vi "Print Initialization Message.vi"(8 "error in (no error)":errorcluster, 11 "Parameters":T1={"Interface Data"={"Name"="", "Unit ID"=0, "Refresh Rate"=0, "Interface Type"=enum."TCP Master", "TCP Settings"={"Address"="", "Port"=0, "Timeout"=0}, "Serial Settings"={"VISA resource name"="", "baud rate"=0, "parity (even)"=0, "flow control (none)"=0, "serial type"=enum."RTU", "Wire Mode"=-1}}, "Modbus Input Groups"=[], "Modbus Output Groups"=[], "error in (no error)"={"status"=FALSE, "code"=0, "source"=""}, "Modbus Input Engine Group Names"=[], "Modbus Output Engine Group Names"=[]} {"Interface Data"."Serial Settings"."Wire Mode" items=["Unknown"=-1, "RS485/Wire4"=0, "RS485/Wire2-EchoDTR"=1, "RS485/Wire2-CtrlDTR"=2, "RS485/Wire2-Auto"=3, "RS232/DTE"=128, "RS232/DCE"=129, "RS232/AUTO"=130]; "Interface Data"."Serial Settings"."parity (even)" items=["None", "Odd", "Even", "Mark", "Space"]; "Interface Data"."Serial Settings"."flow control (none)" items=["None", "XON/XOFF", "RTS/CTS", "XON/XOFF & RTS/CTS", "DTR/DSR", "XON/XOFF & DTR/DSR"]}) -> (0 "error out":errorcluster)   [LabVIEW 2015, in "Modbus Master Engine.lvlib"]
uses:
  Modbus Master Engine.lvlib
  Shared/Device Info.ctl
  Shared/Controls/Interface Type.ctl
  Shared/Controls/Data Model/TCP Settings.ctl
  Shared/Controls/Data Model/Serial Settings.ctl
  Bulk Data Access.ctl
  System Explorer/SubVIs/Modbus Type.ctl
  Shared/Controls/Data Model/Channel.ctl
  <vilib>/NI Veristand/Custom Device API/Custom Device Channel Type.ctl
  Shared/Controls/Data Model/Mapping.ctl
  Shared/Controls/Data Model/DataType.ctl
  <vilib>/NI Veristand/Custom Device API/Custom Device Item Ref.ctl
  <vilib>/NI VeriStand/Custom Device Tools/Custom Device Utility Library/Custom Device Utility Library.lvlib
  Shared/Modbus Master Shared.lvlib
  <vilib>/NI VeriStand/Custom Device API/Custom Device API.lvlib
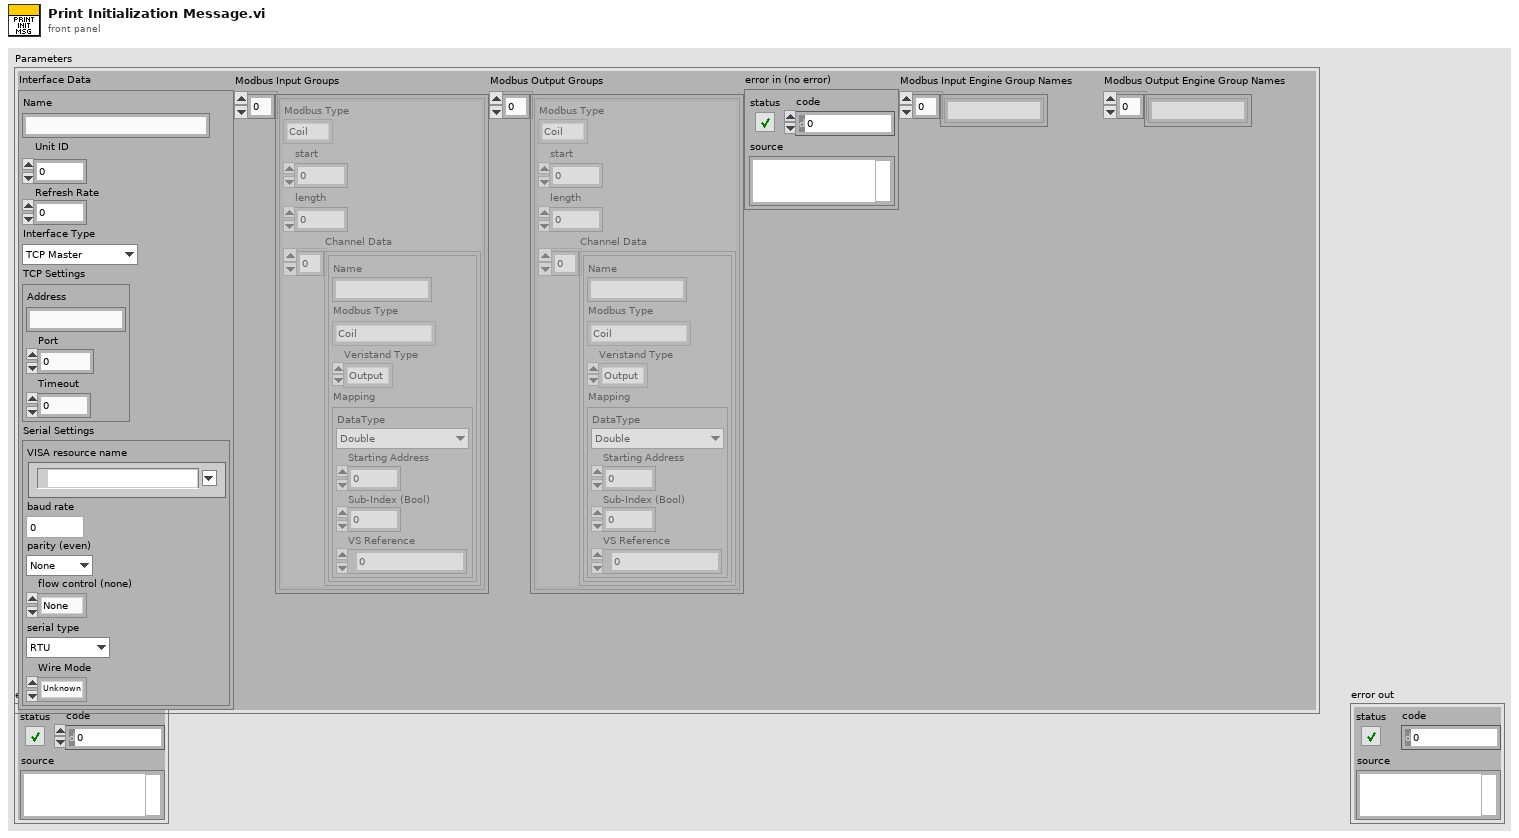
[diagram p1: front panel]
types:
  T1 = typedef "Modbus Master Shared.lvlib/Device Info.ctl" = cluster{"Interface Data":cluster{"Name":string, "Unit ID":u8, "Refresh Rate":i32, "Interface Type":T2, "TCP Settings":T3, "Serial Settings":T4}, "Modbus Input Groups":T5[], "Modbus Output Groups":T5[], "error in (no error)":errorcluster, "Modbus Input Engine Group Names":string[], "Modbus Output Engine Group Names":string[]}
  T2 = typedef "Modbus Master Shared.lvlib/Interface Type.ctl" = enum16{"TCP Master", "Serial Master", "TCP Slave", "Serial Slave"}
  T3 = typedef "Modbus Master Shared.lvlib/TCP Settings.ctl" = cluster{"Address":string, "Port":u16, "Timeout":i32}
  T4 = typedef "Modbus Master Shared.lvlib/Serial Settings.ctl" = cluster{"VISA resource name":refnum<visa-resource-name>, "baud rate":u32, "parity (even)":u16, "flow control (none)":u16, "serial type":enum16{"RTU", "ASCII"}, "Wire Mode":i16}
  T5 = typedef "Modbus Master Shared.lvlib/Bulk Data Access.ctl" = cluster{"Modbus Type":T6, "start":u16, "length":u16, "Channel Data":T7[]}
  T6 = typedef "Modbus Master Shared.lvlib/Modbus Type.ctl" = enum16{"Coil", "Discrete Input", "Holding Register", "Input Register"}
  T7 = typedef "Modbus Master Shared.lvlib/Channel.ctl" = cluster{"Name":string, "Modbus Type":T6, "Veristand Type":T8, "Mapping":T9}
  T8 = typedef "Custom Device API.lvlib/Custom Device Channel Type.ctl" = enum16{"Input", "Output"}
  T9 = typedef "Modbus Master Shared.lvlib/Mapping.ctl" = cluster{"DataType":T10, "Starting Address":u16, "Sub-Index (Bool)":u16, "VS Reference":T11}
  T10 = typedef "Modbus Master Shared.lvlib/DataType.ctl" = enum16{"Double", "Single", "I64", "I32", "I16", "I8", "U64", "U32", "U16", "U8", "Boolean"}
  T11 = typedef "Custom Device API.lvlib/Custom Device Item Ref.ctl" = u64
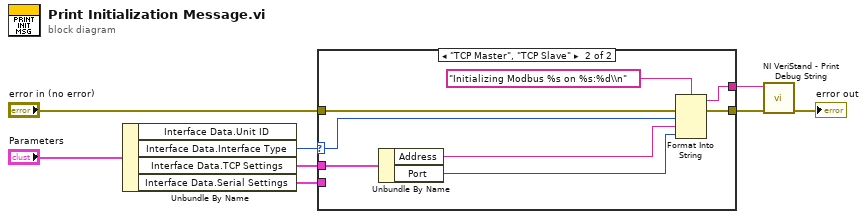
[diagram p0: block diagram]
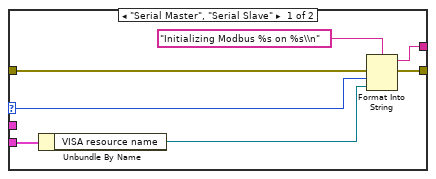
[diagram p2: hidden frame]
diagram:
  n1 = Unbundle By Name("Parameters") -> ("Interface Data.Interface Type"=w5:T2, "Interface Data.TCP Settings"=w7:T3, "Interface Data.Serial Settings"=w6:T4)  [unwired: 1 out]
  n2 = case shown="\"TCP Master\", \"TCP Slave\"" w5 {
    selector: w5 -> [w14 w22]
    tunnel: w6 -> [w13 _]
    tunnel: w7 -> [_ w20]
    tunnel: "error in (no error)" -> [w11 w18]
    tunnel: [w10 w17] -> w2
    tunnel: [w9 w16] -> w3
    frame "Serial Master", "Serial Slave" {
      n3 = Unbundle By Name(w13) -> ("VISA resource name"=w12:refnum<visa-resource-name>)
      n4 = Format Into String(format string="Initializing Modbus %s on %s\\n", error in=w11, w14, w12) -> (resulting string=w9:string, error out=w10:errorcluster)  [unwired: 1 in]
    }
    frame "TCP Master", "TCP Slave" {
      n5 = Unbundle By Name(w20) -> ("Address"=w21:string, "Port"=w19:u16)
      n6 = Format Into String(format string="Initializing Modbus %s on %s:%d\\n", error in=w18, w22, w21, w19) -> (resulting string=w16:string, error out=w17:errorcluster)  [unwired: 1 in]
    }
  }
  n7 = call <vilib>:"NI VeriStand - Print Debug String.vi"("error in (no error)"=w2, "Message"=w3) -> ("error out"=→"error out":errorcluster)  [unwired: 9 in]
